vi "Create Last Temperature Entry.vi"(8 "error in":errorcluster, 10 "Channel":string, 11 "Thermometer DAQmx RTD Cont CFG in":refnum<class "Thermometer DAQmx TC Cont CFG.lvclass">) -> (0 "error out":errorcluster, 3 "Thermometer DAQmx RTD Cont CFG out":refnum<class "Thermometer DAQmx TC Cont CFG.lvclass">)   [LabVIEW 2024, in "Thermometer DAQmx TC Cont CFG.lvclass"]
uses:
  Thermometer DAQmx TC Cont CFG.lvclass
  Thermometer DAQmx TC Cont CFG.lvclass/Thermometer DAQmx TC Cont CFG.ctl
  <vilib>/Utility/miscctls.llb/LVMapReplaceAction.ctl
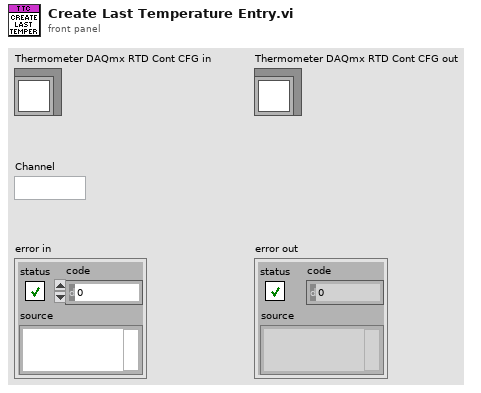
[diagram p1: front panel]
types:
  T1 = typedef "LVMapReplaceAction.ctl" = enum32{"Modify Entry only if found", "Add or Modify Entry", "Delete Entry"}
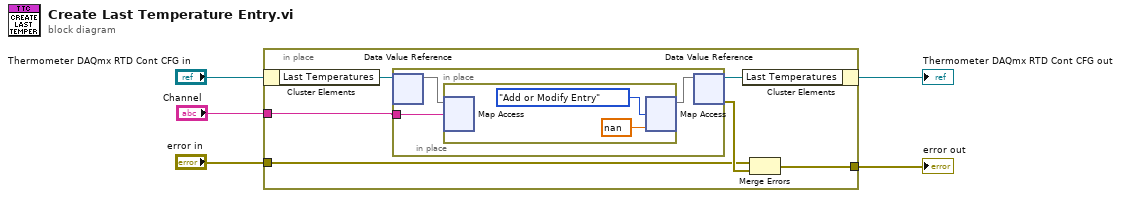
[diagram p0: block diagram]
diagram:
  n1 = in-place {
    in-place-border: "Channel" -> [w10]
    in-place-border: "error in" -> [w8]
    in-place-border: [w7] -> w4
    n2 = in-place-cluster #1("Thermometer DAQmx RTD Cont CFG in") -> ("Last Temperatures"=w11:refnum<data-value>)
    n3 = in-place {
      in-place-border: w10 -> [w13]
      n4 = in-place-dvr #2(w11) -> (w14:map{string, dbl})  [unwired: 1 out]
      n5 = in-place {
        n6 = in-place-map #3(w14, w13) -> ()  [unwired: 1 in, 2 out]
        n7 = in-place-map #3(nan, LVMapReplaceAction."Add or Modify Entry" ("action")) -> (w12:map{string, dbl})  [unwired: 2 out]
      }
      n8 = in-place-dvr #2(w12) -> (w6:refnum<data-value>, w9:errorcluster)
    }
    n9 = in-place-cluster #1("Last Temperatures"=w6) -> (→"Thermometer DAQmx RTD Cont CFG out":refnum<class "Thermometer DAQmx TC Cont CFG.lvclass">)
    n10 = Merge Errors(w8, w9) -> (w7:errorcluster)
  }
  "error out" <- w4
